vi "5_2 Infrared Based Proximity Detection.vi"() -> ()   [LabVIEW 2025]
panel:
  in  "stop":bool
  out "Status Indicator":bool
  out "Message":string
  in  "Voltage across photo Transistor":dbl
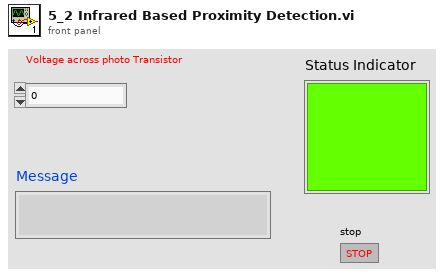
[diagram p1: front panel]
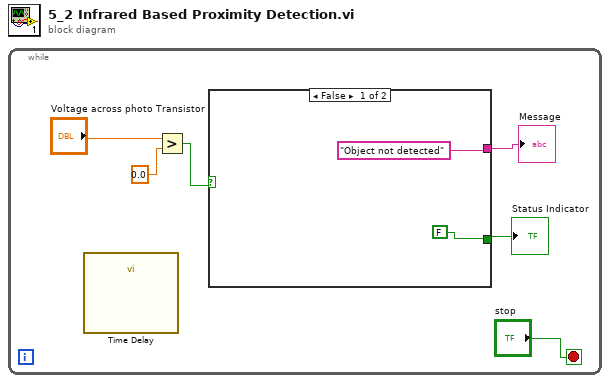
[diagram p0: block diagram]
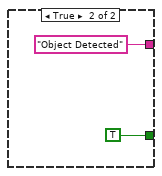
[diagram p2: hidden frame]
diagram:
  n1 = while {
    stop <- "stop" stop-if-true
    n2 = call "Time Delay"() -> ()  [unwired: 11 in, 1 out]
    n3 = Greater?(x="Voltage across photo Transistor", y=0.0) -> (0:w1:bool)
    n4 = case shown="False" w1 {
      tunnel: ["Object not detected" "Object Detected"] -> w4
      tunnel: [FALSE TRUE] -> w3
      frame False {
      }
      frame True {
      }
    }
    "Message" <- w4
    "Status Indicator" <- w3
  }
